vi "AllGaugePressures.vi"(8 "error in (no error)":errorcluster, 11 "VacSys in":refnum<class "VacSys.lvclass">) -> (0 "error out":errorcluster, 2 "Pressures":dbl[](array[numeric]), 3 "VacSys out":refnum<class "VacSys.lvclass">)   [LabVIEW 2016, in "VacSys.lvclass"]
uses:
  VacSys.lvclass
  VacSys.lvclass/VacSys.ctl
  Interfaces/IGauge/IGauge.lvclass
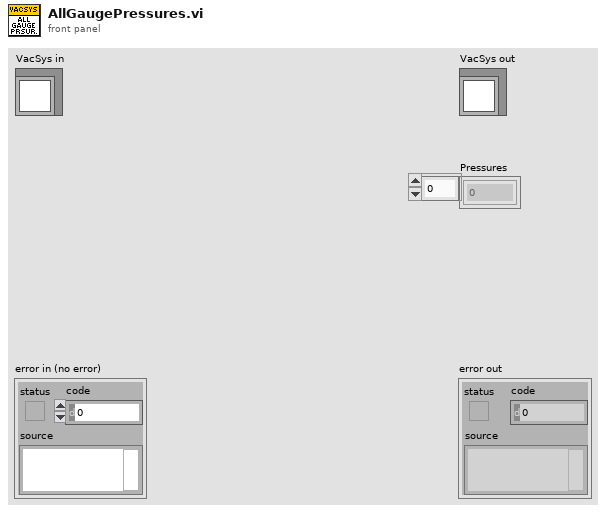
[diagram p1: front panel]
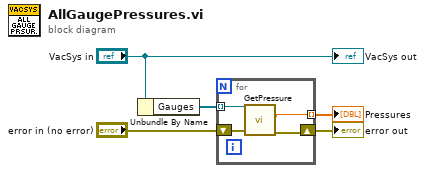
[diagram p0: block diagram]
diagram:
  n1 = Unbundle By Name("VacSys in") -> ("Gauges"=w4:refnum<class "IGauge.lvclass">[])
  n2 = for {
    tunnel: w4 -> [w9] mode=indexing
    shift-right: [w6] -> w1
    shift-left: "error in (no error)" -> [w8]
    tunnel: [w7] -> w3 mode=indexing
    n3 = call-dynamic "GetPressure.vi"("error in (no error)"=w8, "IGauge in"=w9) -> ("error out"=w6:errorcluster, "Pressure (mbar)"=w7:dbl)  [unwired: 7 in, 1 out]
  }
  "error out" <- w1
  "Pressures" <- w3
  "VacSys out" <- "VacSys in"
